vi "DCA Compute T-Attenuation.vi"(1 "Measurement Values":T1) -> (0 "T-Attenuation":dbl)   [LabVIEW 2011]
uses:
  TypeDefs/DCA Measurement Values.ctl
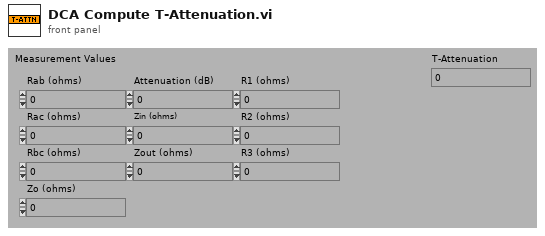
[diagram p1: front panel]
types:
  T1 = typedef "DCA Measurement Values.ctl" = cluster{"Rab (ohms)":dbl, "Rac (ohms)":dbl, "Rbc (ohms)":dbl, "Zo (ohms)":dbl, "Attenuation (dB)":dbl, "Zin (ohms)":dbl, "Zout (ohms)":dbl, "R1 (ohms)":dbl, "R2 (ohms)":dbl, "R3 (ohms)":dbl}
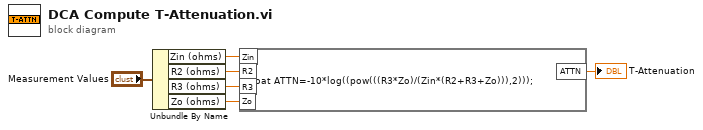
[diagram p0: block diagram]
diagram:
  n1 = Unbundle By Name("Measurement Values") -> ("Zin (ohms)"=w5:dbl, "R2 (ohms)"=w4:dbl, "R3 (ohms)"=w3:dbl, "Zo (ohms)"=w1:dbl)
  n2 = formula code="float ATTN=-10*log((pow(((R3*Zo)/(Zin*(R2+R3+Zo))),2)));"("Zin"=w5, "R2"=w4, "R3"=w3, "Zo"=w1) -> ("ATTN"=→"T-Attenuation":dbl)
